vi "FTW-Container-Value-DBL.vi"(0 "JSON":refnum<class "FTW-Container.lvclass">, 11 "error in":errorcluster) -> (4 "JSON out":refnum<class "FTW-Container.lvclass">, 8 "Value":dbl, 15 "error out":errorcluster)   [LabVIEW 2015, in "FTW-Container.lvclass"]
uses:
  FTW-Container.lvclass
panel:
  # "Inputs"
  # "Outputs"
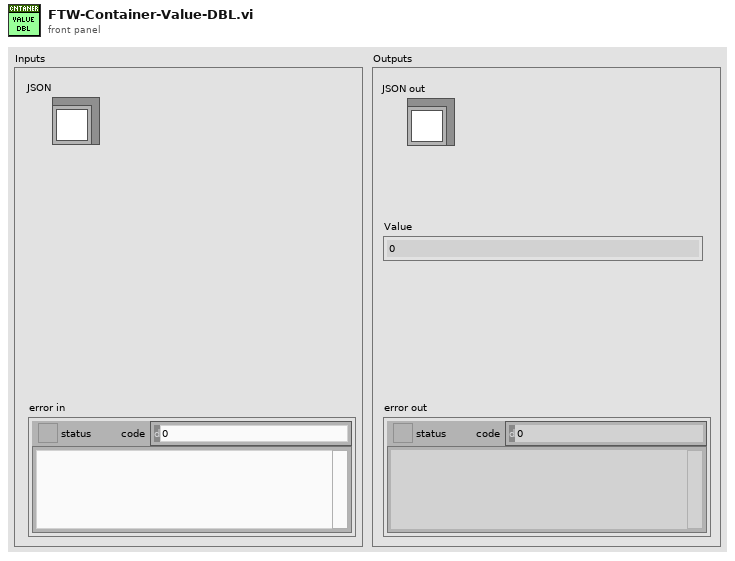
[diagram p1: front panel]
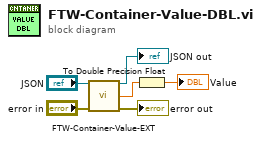
[diagram p0: block diagram]
diagram:
  n1 = call "FTW-Container-Value-EXT.vi"("JSON"="JSON", "error in"="error in") -> ("JSON out"=→"JSON out":refnum<class "FTW-Container.lvclass">, "Value"=w4:ext, "error out"=→"error out":errorcluster)  [unwired: 11 in]
  n2 = To Double Precision Float(number=w4) -> (double precision float=→"Value":dbl)
